vi "Graph_readCursorIndex.vi"(1 "existing cursor\nname":string, 2 "Cursor List":T1(array[cluster])) -> (0 "cursor index":i32)   [LabVIEW 2010]
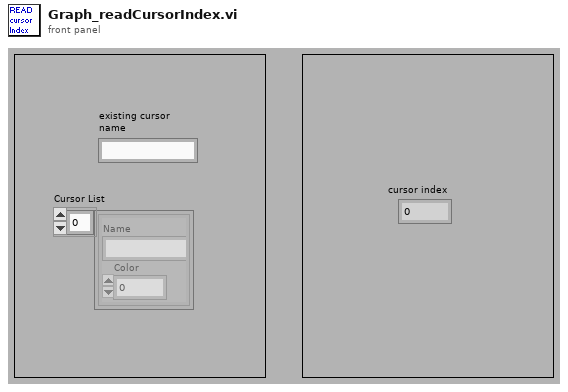
[diagram p1: front panel]
types:
  T1 = cluster{"Name":string, "Color":u32, "Style":u8, "Point Style":u8, "Name Visible":bool, "Allow Drag":bool, "Cursor Mode":u32, "Plot":i32, "Index":i32, "Position":cluster{"X":dbl, "Y":dbl}, "X Scale":u32, "Y Scale":u32, "Watch Plots":i32[], "Watch All Plots":bool, "Plot Area":i32, "Label Offset":cluster{"X":dbl, "Y":dbl}}[]
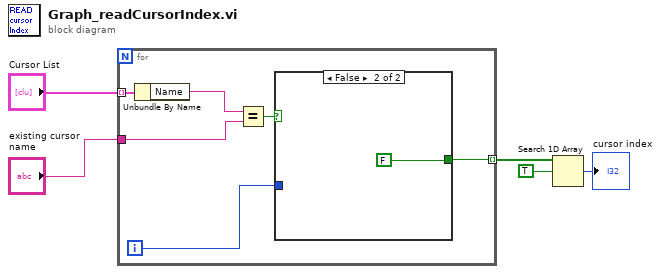
[diagram p0: block diagram]
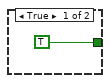
[diagram p2: hidden frame]
diagram:
  n1 = for {
    tunnel: "Cursor List" -> [w11] mode=indexing
    tunnel: "existing cursor\nname" -> [w8]
    tunnel: [w6] -> w3 mode=indexing
    i -> [w9]
    n2 = Unbundle By Name(w11) -> ("Name"=w7:string)
    n3 = Equal?(x=w7, y=w8) -> (x = y?=w10:bool)
    n4 = case shown="False" w10 {
      tunnel: w9 -> [_ _]
      tunnel: [TRUE FALSE] -> w6
      frame True {
      }
      frame False {
      }
    }
  }
  n5 = Search 1D Array(1D array=w3, element=TRUE) -> (index of element=→"cursor index":i32)  [unwired: 1 in]
